vi "Part-22-Generating-Signal.vi"() -> ()   [LabVIEW 2015]
uses:
  <userlib>/TripleDisplayX.llb/TripleDisplay.xctl
panel:
  in  "sampling info 3":cluster{"Fs":dbl, "#s":dbl}={"Fs"=1000.0, "#s"=1000.0} {"Fs" format="%.2p"}
  in  "sampling info 2":cluster{"Fs":dbl, "#s":dbl}={"Fs"=1000.0, "#s"=1000.0} {"Fs" format="%.2p"}
  in  "sampling info":cluster{"Fs":dbl, "#s":dbl}={"Fs"=1000.0, "#s"=1000.0} {"Fs" format="%.2p"}
  in  "signal type 3":T1(ring)
  in  "frequency 3":dbl=10.0 format="%0.2p"
  out "TripleDisplay 3":waveform(dbl)(xcontrol)
  out "TripleDisplay 2":waveform(dbl)(xcontrol)
  in  "phase 2":dbl format="%.2p"
  in  "amplitude 2":dbl=1.0 format="%0.2p"
  in  "frequency 2":dbl=10.0 format="%0.2p"
  in  "signal type 2":T1(ring)
  in  "signal type":T1(ring)
  in  "phase":dbl format="%.2p"
  in  "amplitude":dbl=1.0 format="%0.2p"
  in  "frequency":dbl=10.0 format="%0.2p"
  out "TripleDisplay":waveform(dbl)(xcontrol)
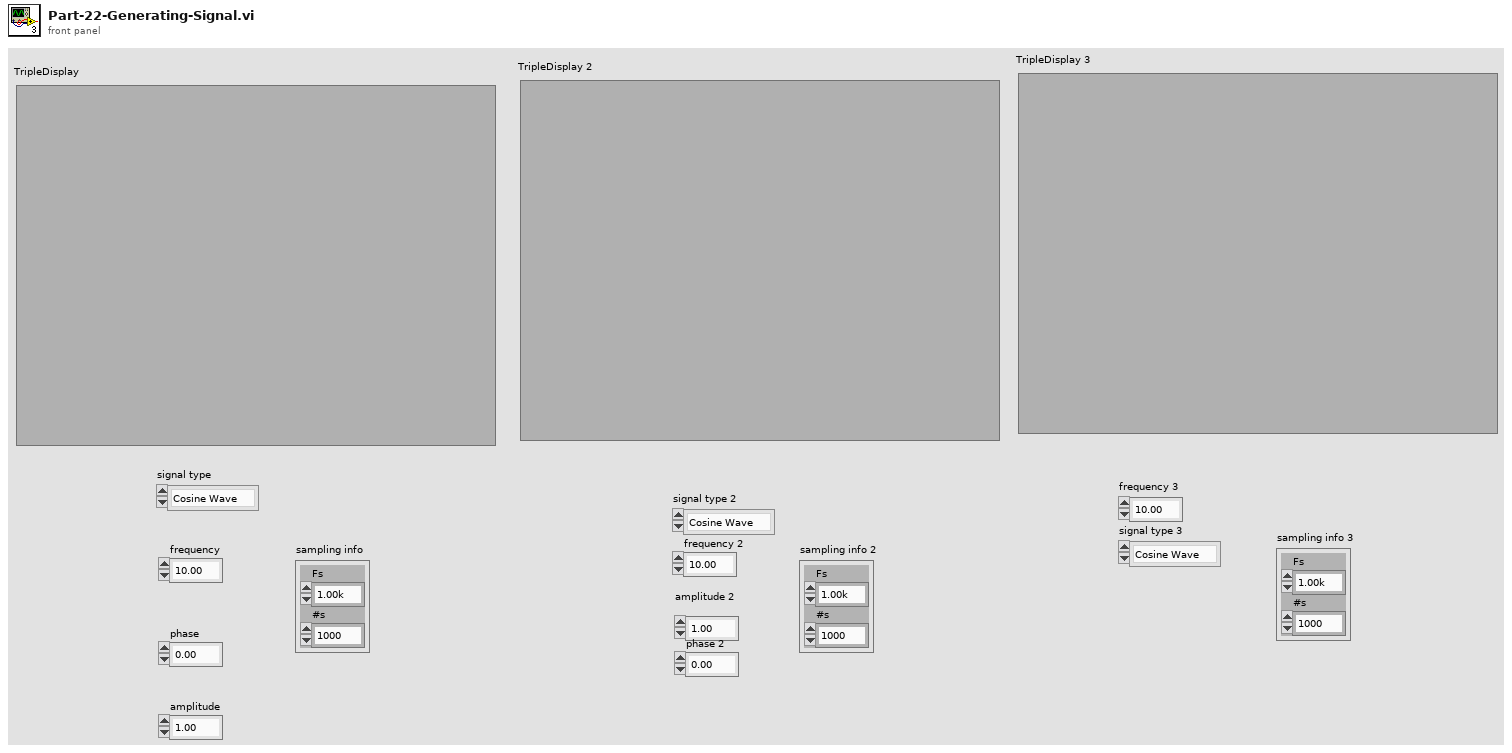
[diagram p1: front panel]
types:
  T1 = enum16{"Cosine Wave", "Sine Wave", "Triangle Wave", "Square Wave", "Sawtooth Wave"}
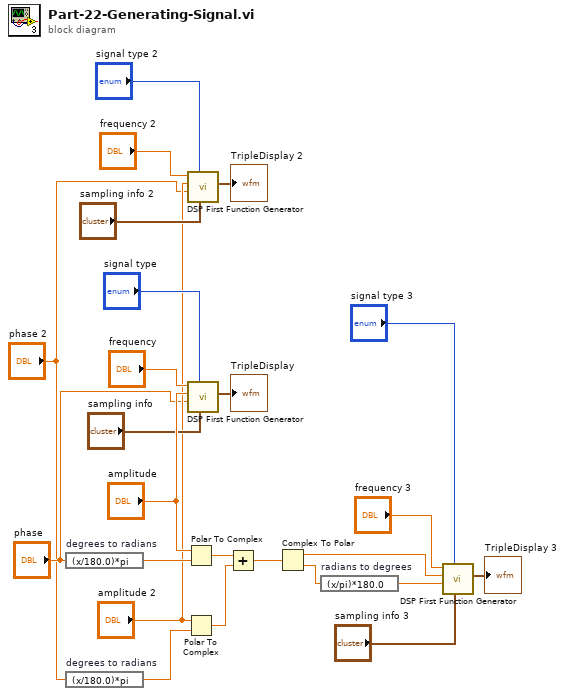
[diagram p0: block diagram]
diagram:
  n1 = expression code="(x/180.0)*pi" "degrees to radians"("phase") -> (w4:dbl)
  n2 = expression code="(x/180.0)*pi" "degrees to radians"("phase 2") -> (w5:dbl)
  n3 = Polar To Complex(1:w4, 2:"amplitude") -> (0:w17:cdb)
  n4 = Polar To Complex(1:w5, 2:"amplitude 2") -> (0:w16:cdb)
  n5 = call <userlib>:"DSP First Function Generator.vi"("sampling info"="sampling info 2", "signal type"="signal type 2", "phase"="phase 2", "amplitude"="amplitude 2", "frequency"="frequency 2") -> ("signal out"=→"TripleDisplay 2":waveform(dbl))  [unwired: 4 in, 2 out]
  n6 = call <userlib>:"DSP First Function Generator.vi"("sampling info"="sampling info", "signal type"="signal type", "phase"="phase", "amplitude"="amplitude", "frequency"="frequency") -> ("signal out"=→"TripleDisplay":waveform(dbl))  [unwired: 4 in, 2 out]
  n7 = Add(x=w17, y=w16) -> (x+y=w15:cdb)
  n8 = Complex To Polar(r * e^(i*theta)=w15) -> (r=w14:dbl, theta=w13:dbl)
  n9 = expression code="(x/pi)*180.0" "radians to degrees"(w13) -> (w6:dbl)
  n10 = call <userlib>:"DSP First Function Generator.vi"("sampling info"="sampling info 3", "signal type"="signal type 3", "phase"=w6, "amplitude"=w14, "frequency"="frequency 3") -> ("signal out"=→"TripleDisplay 3":waveform(dbl))  [unwired: 4 in, 2 out]
